vi "FormulaNodeAddIO.vi"(0 "__args":T1) -> (1 "__return":i32, 2 "__errStatus":bool, 3 "__errCode":i32, 4 "__errSource":string)   [LabVIEW 2013]
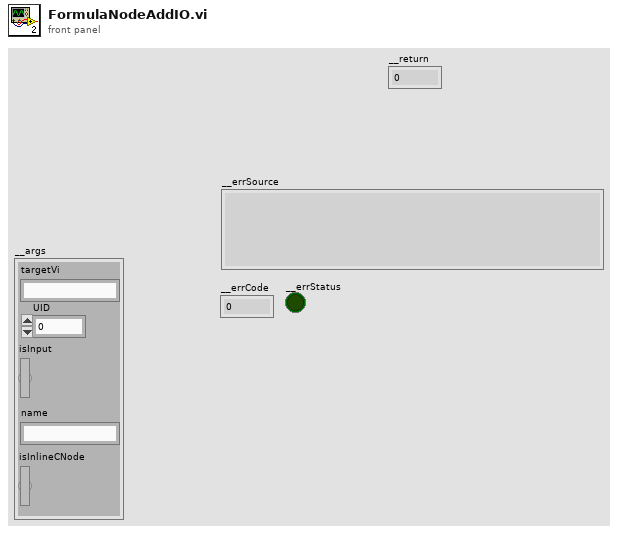
[diagram p1: front panel]
types:
  T1 = cluster{"targetVi":string, "UID":i32, "isInput":bool, "name":string, "isInlineCNode":bool}
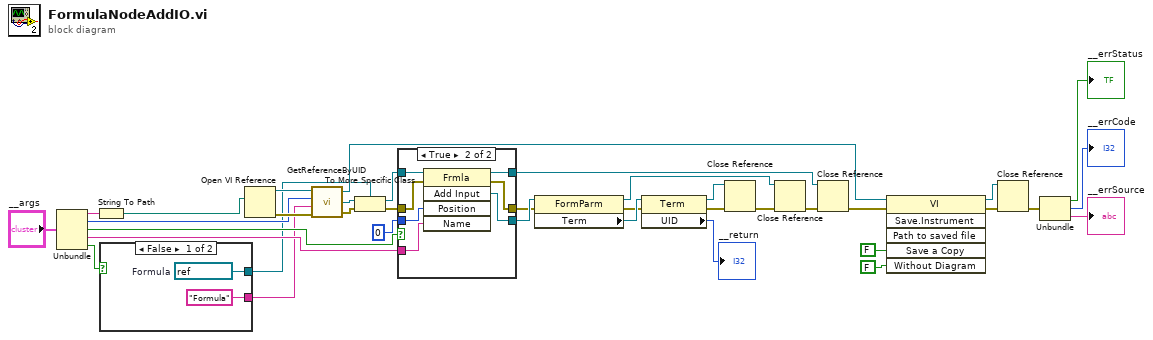
[diagram p0: block diagram]
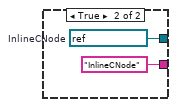
[diagram p2: hidden frame]
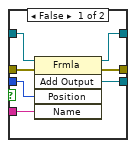
[diagram p3: hidden frame]
diagram:
  n1 = Unbundle("__args") -> ("targetVi"=w31:string, "UID"=w29:i32, "isInput"=w24:bool, "name"=w22:string, "isInlineCNode"=w3:bool)
  n2 = String To Path(string=w31) -> (path=w33:path)
  n3 = case shown="False" w3 {
    tunnel: [w39 w41] -> w2
    tunnel: ["Formula" ("objectClass") "InlineCNode" ("objectClass")] -> w1
    frame False {
      w39 = refnum<vi> refnum  # Formula
    }
    frame True {
      w41 = refnum<vi> refnum  # InlineCNode
    }
  }
  n4 = Open VI Reference(vi path=w33) -> (vi reference=w30:refnum<vi>, error out=w32:errorcluster)  [unwired: 5 in]
  n5 = call "GetReferenceByUID.vi"("error in (no error)"=w32, "objectClass"=w1, "UID"=w29, "targetVI"=w30) -> ("error out"=w28:errorcluster, "refNum"=w27:refnum<vi>, "dup targetVI"=w7:refnum<vi>)
  n6 = To More Specific Class(target class=w2, reference=w27, error in=w28) -> (specific class reference=w26:refnum<vi>, error out=w25:errorcluster)
  n7 = case shown="True" w24 {
    tunnel: w26 -> [w48 w55]
    tunnel: w25 -> [w47 w54]
    tunnel: [w46 w52] -> w23
    tunnel: w22 -> [w45 w53]
    tunnel: [w43 w51] -> w21
    tunnel: [w44 w50] -> w16
    tunnel: u32 0 ("Position") -> [w42 w49]
    frame False {
      n8 = invoke class="Frmla" method="Add Output"(reference=w48, error in=w47, "Position"=w42, "Name"=w45) -> (reference out=w46:refnum<vi>, error out=w44:errorcluster, "Add Output"=w43:refnum<vi>)  [unwired: 1 in, 2 out]
    }
    frame True {
      n9 = invoke class="Frmla" method="Add Input"(reference=w55, error in=w54, "Position"=w49, "Name"=w53) -> (reference out=w52:refnum<vi>, error out=w50:errorcluster, "Add Input"=w51:refnum<vi>)  [unwired: 1 in, 2 out]
    }
  }
  n10 = property class="FormParm"(reference=w21, error in=w16) -> (reference out=w10:refnum<vi>, error out=w15:errorcluster, "Term"=w18:refnum<vi>)
  n11 = property class="Term"(reference=w18, error in=w15) -> (reference out=w11:refnum<vi>, error out=w12:errorcluster, "UID"=→"__return":i32)
  n12 = Close Reference(reference=w11, error in (no error)=w12) -> (error out=w14:errorcluster)
  n13 = Close Reference(reference=w10, error in (no error)=w14) -> (error out=w13:errorcluster)
  n14 = Close Reference(reference=w23, error in (no error)=w13) -> (error out=w6:errorcluster)
  n15 = invoke class="VI" method="Save.Instrument"(reference=w7, error in=w6, "Save a Copy"=FALSE, "Without Diagram"=FALSE) -> (reference out=w4:refnum<vi>, error out=w5:errorcluster)  [unwired: 2 in, 4 out]
  n16 = Close Reference(reference=w4, error in (no error)=w5) -> (error out=w20:errorcluster)
  n17 = Unbundle(w20) -> ("status"=→"__errStatus":bool, "code"=→"__errCode":i32, "source"=→"__errSource":string)
